vi "Set Properties from Cluster.vi"(8 "error in":errorcluster, 10 "Variant Cluster":variant, 11 "item ref in":T1 format="%.0x") -> (0 "error out":errorcluster, 3 "item ref out":T1 format="%.0x")   [LabVIEW 2020, in "AIM ARINC 664 Scripting.lvlib"]
doc: "Set the parameters cluster into the system definition, separating each element by name in cluster.\n\nBe sure that cluster element names are matching Veristand Property names.\n\nDo not pass clusters of clusters or array of cluster as inputs to this VI. It only works with plain clusters."
uses:
  AIM ARINC 664 Scripting.lvlib
  <vilib>/NI VeriStand/Custom Device API/Custom Device Item Ref.ctl
  <vilib>/NI VeriStand/Custom Device API/Set Item Property (U32).vi
  <vilib>/NI VeriStand/Custom Device API/Set Item Property (U16).vi
  <vilib>/NI VeriStand/Custom Device API/Set Item Property (Double).vi
  <vilib>/NI VeriStand/Custom Device API/Set Item Property (I32).vi
  <vilib>/NI VeriStand/Custom Device API/Set Item Property (String).vi
  <vilib>/NI VeriStand/Custom Device API/Set Item Property (Path).vi
  <vilib>/NI VeriStand/Custom Device API/Set Item Property (Boolean).vi
  <vilib>/NI VeriStand/Custom Device API/Custom Device API.lvlib
  <vilib>/Utility/Data Type/NI_Data Type.lvlib
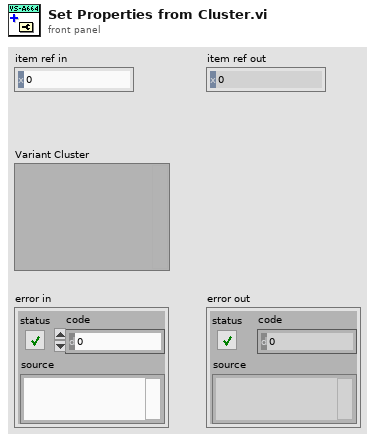
[diagram p1: front panel]
types:
  T1 = typedef "Custom Device API.lvlib/Custom Device Item Ref.ctl" = u64
  T2 = typedef "NI_Data Type.lvlib/Data Type.ctl" = enum8{"Invalid Type", "Void", "I8", "I16", "I32", "I64", "U8", "U16", "U32", "U64", "Single Float", "Double Float", "Extended Float", "Single Complex", "Double Complex", "Extended Complex", "Enum U8", "Enum U16", "Enum U32", "Enum U64", "Single Float With Unit", "Double Float With Unit", "Extended Float With Unit", "Single Complex with Unit", "Double Complex with Unit", "Extended Complex with Unit", "Boolean", "String", "Path", "Picture", "Tag", "Array", "Cluster", "Variant", "LV Variant", "Waveform", "Timestamp", "Digital Waveform", "Digital Data", "ExpressData", "Refnum", "External Data", "VI", "Poly VI", "LabVIEW Class Instance", "Fixed Point", "Set Collection", "Map Collection"}
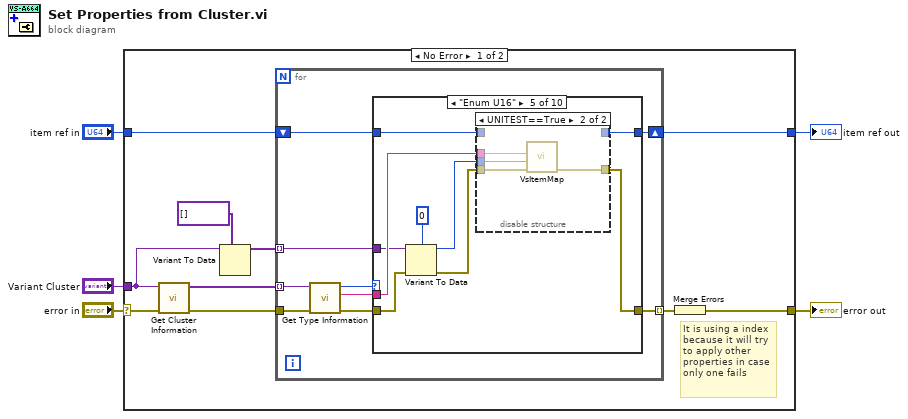
[diagram p0: block diagram]
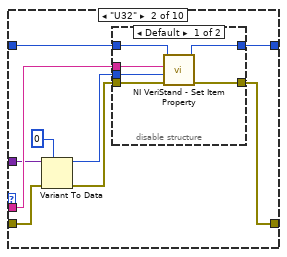
[diagram p3: hidden frame]
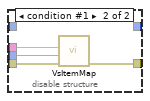
[diagram p4: hidden frame]
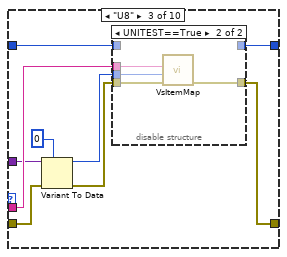
[diagram p5: hidden frame]
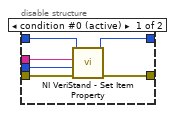
[diagram p6: hidden frame]
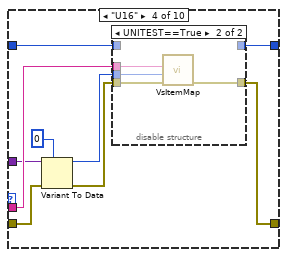
[diagram p7: hidden frame]
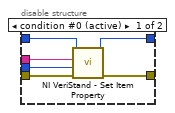
[diagram p8: hidden frame]
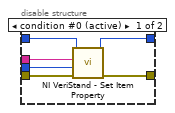
[diagram p9: hidden frame]
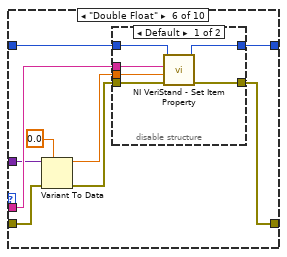
[diagram p10: hidden frame]
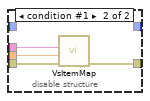
[diagram p11: hidden frame]
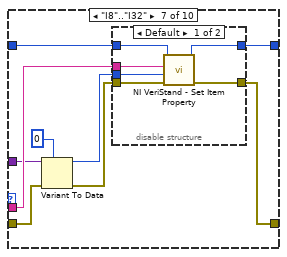
[diagram p12: hidden frame]
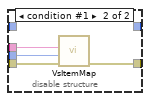
[diagram p13: hidden frame]
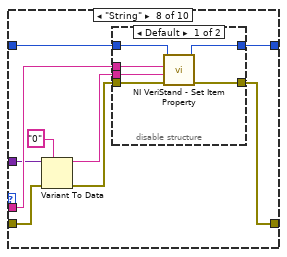
[diagram p14: hidden frame]
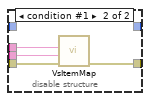
[diagram p15: hidden frame]
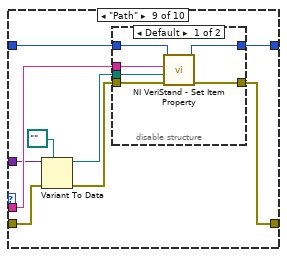
[diagram p16: hidden frame]
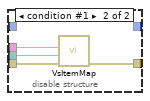
[diagram p17: hidden frame]
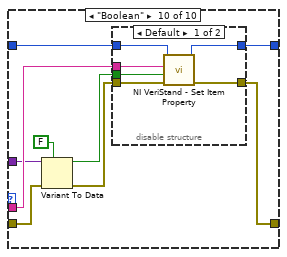
[diagram p18: hidden frame]
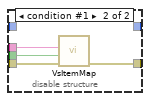
[diagram p19: hidden frame]
diagram:
  n1 = case shown="No Error" "error in" {
    selector: "error in" -> [w6 w190]
    tunnel: "item ref in" -> [w15 w189]
    tunnel: [w13 w189] -> w4
    tunnel: "Variant Cluster" -> [w8 _]
    tunnel: [w7 w190] -> w2
    frame No Error {
      # "It is using a index\nbecause it will try\nto apply other\nproperties in case\nonly one fails"
      n2 = call <vilib>:"Get Cluster Information.vi"("error in (no error)"=w6, "variant"=w8) -> ("error out"=w11:errorcluster, "cluster elements"=w12:variant[])  [unwired: 8 in]
      n3 = Variant To Data(type=variant[] [], Variant=w8) -> (data=w10:variant[])  [unwired: 1 in, 1 out]
      n4 = for {
        tunnel: w12 -> [w24] mode=indexing
        shift-right: [w20] -> w13
        shift-left: w15 -> [w21]
        tunnel: w10 -> [w16] mode=indexing
        tunnel: w11 -> [w23]
        tunnel: [w17] -> w14 mode=indexing
        n5 = call <vilib>:"Get Type Information.vi"("error in (no error)"=w23, "variant"=w24) -> ("error out"=w18:errorcluster, "name"=w22:string, "type"=w19:T2)  [unwired: 5 in, 2 out]
        n6 = case shown="\"Enum U16\"" w19 {
          tunnel: w22 -> [_ w35 w53 w71 w89 w107 w125 w143 w161 w179]
          tunnel: w21 -> [w26 w34 w52 w70 w88 w106 w124 w142 w160 w178]
          tunnel: [w26 w33 w51 w69 w87 w105 w123 w141 w159 w177] -> w20
          tunnel: w18 -> [w25 w28 w46 w64 w83 w100 w118 w136 w154 w173]
          tunnel: [w25 w32 w50 w68 w86 w104 w122 w140 w158 w176] -> w17
          tunnel: w16 -> [_ w31 w49 w67 w85 w103 w121 w139 w157 w175]
          frame "Invalid Type", Default {
          }
          frame "U32" {
            n7 = Variant To Data(error in=w28, type=u32 0, Variant=w31) -> (data=w30:u32, error out=w27:errorcluster)
            n8 = disable-structure shown="Default" {
              disable-tunnel: w35 -> [w41 w44]
              disable-tunnel: w34 -> [w40 _]
              disable-tunnel: [w39 _] -> w33
              disable-tunnel: [w38 w42] -> w32
              disable-tunnel: w30 -> [w37 w43]
              disable-tunnel: w27 -> [w36 w42]
              frame condition #0 (active) {
                n9 = call-poly <vilib>:"NI VeriStand - Set Item Property.vi"("error in (no error)"=w36, "Value"=w37, "Property Name"=w41, "Item Ref in"=w40) -> ("error out"=w38:errorcluster, "Item Ref out"=w39:T1)  [unwired: 5 in, 1 out]
              }
              frame condition #1 {
                n10 = call "VsItemMap.vi"("Variant"=w43, "name"=w44) -> ()  [unwired: 9 in, 1 out]
              }
            }
          }
          frame "U8" {
            n11 = Variant To Data(error in=w46, type=u8 0, Variant=w49) -> (data=w48:u8, error out=w45:errorcluster)
            n12 = disable-structure shown="UNITEST==True" {
              disable-tunnel: w53 -> [w59 w62]
              disable-tunnel: w52 -> [w58 _]
              disable-tunnel: [w57 _] -> w51
              disable-tunnel: [w56 w60] -> w50
              disable-tunnel: w48 -> [w55 w61]
              disable-tunnel: w45 -> [w54 w60]
              frame condition #0 (active) {
                n13 = call-poly <vilib>:"NI VeriStand - Set Item Property.vi"("error in (no error)"=w54, "Value"=w55, "Property Name"=w59, "Item Ref in"=w58) -> ("error out"=w56:errorcluster, "Item Ref out"=w57:T1)  [unwired: 5 in, 1 out]
              }
              frame condition #1 {
                n14 = call "VsItemMap.vi"("Variant"=w61, "name"=w62) -> ()  [unwired: 9 in, 1 out]
              }
            }
          }
          frame "U16" {
            n15 = Variant To Data(error in=w64, type=u16 0, Variant=w67) -> (data=w66:u16, error out=w63:errorcluster)
            n16 = disable-structure shown="UNITEST==True" {
              disable-tunnel: w71 -> [w77 w80]
              disable-tunnel: w70 -> [w76 _]
              disable-tunnel: [w75 _] -> w69
              disable-tunnel: [w74 w78] -> w68
              disable-tunnel: w66 -> [w73 w79]
              disable-tunnel: w63 -> [w72 w78]
              frame condition #0 (active) {
                n17 = call-poly <vilib>:"NI VeriStand - Set Item Property.vi"("error in (no error)"=w72, "Value"=w73, "Property Name"=w77, "Item Ref in"=w76) -> ("error out"=w74:errorcluster, "Item Ref out"=w75:T1)  [unwired: 5 in, 1 out]
              }
              frame condition #1 {
                n18 = call "VsItemMap.vi"("Variant"=w79, "name"=w80) -> ()  [unwired: 9 in, 1 out]
              }
            }
          }
          frame "Enum U16" {
            n19 = Variant To Data(error in=w83, type=u16 0, Variant=w85) -> (data=w84:u16, error out=w82:errorcluster)
            n20 = disable-structure shown="UNITEST==True" {
              disable-tunnel: w89 -> [w95 w98]
              disable-tunnel: w88 -> [w94 _]
              disable-tunnel: [w93 _] -> w87
              disable-tunnel: [w92 w96] -> w86
              disable-tunnel: w84 -> [w91 w97]
              disable-tunnel: w82 -> [w90 w96]
              frame condition #0 (active) {
                n21 = call-poly <vilib>:"NI VeriStand - Set Item Property.vi"("error in (no error)"=w90, "Value"=w91, "Property Name"=w95, "Item Ref in"=w94) -> ("error out"=w92:errorcluster, "Item Ref out"=w93:T1)  [unwired: 5 in, 1 out]
              }
              frame condition #1 {
                n22 = call "VsItemMap.vi"("Variant"=w97, "name"=w98) -> ()  [unwired: 9 in, 1 out]
              }
            }
          }
          frame "Double Float" {
            n23 = Variant To Data(error in=w100, type=0.0, Variant=w103) -> (data=w102:dbl, error out=w99:errorcluster)
            n24 = disable-structure shown="Default" {
              disable-tunnel: w107 -> [w113 w116]
              disable-tunnel: w106 -> [w112 _]
              disable-tunnel: [w111 _] -> w105
              disable-tunnel: [w110 w114] -> w104
              disable-tunnel: w102 -> [w109 w115]
              disable-tunnel: w99 -> [w108 w114]
              frame condition #0 (active) {
                n25 = call-poly <vilib>:"NI VeriStand - Set Item Property.vi"("error in (no error)"=w108, "Value"=w109, "Property Name"=w113, "Item Ref in"=w112) -> ("error out"=w110:errorcluster, "Item Ref out"=w111:T1)  [unwired: 5 in, 1 out]
              }
              frame condition #1 {
                n26 = call "VsItemMap.vi"("Variant"=w115, "name"=w116) -> ()  [unwired: 9 in, 1 out]
              }
            }
          }
          frame "I8".."I32" {
            n27 = Variant To Data(error in=w118, type=0, Variant=w121) -> (data=w120:i32, error out=w117:errorcluster)
            n28 = disable-structure shown="Default" {
              disable-tunnel: w125 -> [w131 w134]
              disable-tunnel: w124 -> [w130 _]
              disable-tunnel: [w129 _] -> w123
              disable-tunnel: [w128 w132] -> w122
              disable-tunnel: w120 -> [w127 w133]
              disable-tunnel: w117 -> [w126 w132]
              frame condition #0 (active) {
                n29 = call-poly <vilib>:"NI VeriStand - Set Item Property.vi"("error in (no error)"=w126, "Value"=w127, "Property Name"=w131, "Item Ref in"=w130) -> ("error out"=w128:errorcluster, "Item Ref out"=w129:T1)  [unwired: 5 in, 1 out]
              }
              frame condition #1 {
                n30 = call "VsItemMap.vi"("Variant"=w133, "name"=w134) -> ()  [unwired: 9 in, 1 out]
              }
            }
          }
          frame "String" {
            n31 = Variant To Data(error in=w136, type="0", Variant=w139) -> (data=w138:string, error out=w135:errorcluster)
            n32 = disable-structure shown="Default" {
              disable-tunnel: w143 -> [w149 w152]
              disable-tunnel: w142 -> [w148 _]
              disable-tunnel: [w147 _] -> w141
              disable-tunnel: [w146 w150] -> w140
              disable-tunnel: w138 -> [w145 w151]
              disable-tunnel: w135 -> [w144 w150]
              frame condition #0 (active) {
                n33 = call-poly <vilib>:"NI VeriStand - Set Item Property.vi"("error in (no error)"=w144, "Value"=w145, "Property Name"=w149, "Item Ref in"=w148) -> ("error out"=w146:errorcluster, "Item Ref out"=w147:T1)  [unwired: 5 in, 1 out]
              }
              frame condition #1 {
                n34 = call "VsItemMap.vi"("Variant"=w151, "name"=w152) -> ()  [unwired: 9 in, 1 out]
              }
            }
          }
          frame "Path" {
            n35 = Variant To Data(error in=w154, type=path "", Variant=w157) -> (data=w156:path, error out=w153:errorcluster)
            n36 = disable-structure shown="Default" {
              disable-tunnel: w161 -> [w167 w170]
              disable-tunnel: w160 -> [w166 _]
              disable-tunnel: [w165 _] -> w159
              disable-tunnel: [w164 w168] -> w158
              disable-tunnel: w156 -> [w163 w169]
              disable-tunnel: w153 -> [w162 w168]
              frame condition #0 (active) {
                n37 = call-poly <vilib>:"NI VeriStand - Set Item Property.vi"("error in (no error)"=w162, "Value"=w163, "Property Name"=w167, "Item Ref in"=w166) -> ("error out"=w164:errorcluster, "Item Ref out"=w165:T1)  [unwired: 5 in, 1 out]
              }
              frame condition #1 {
                n38 = call "VsItemMap.vi"("Variant"=w169, "name"=w170) -> ()  [unwired: 9 in, 1 out]
              }
            }
          }
          frame "Boolean" {
            n39 = Variant To Data(error in=w173, type=FALSE, Variant=w175) -> (data=w174:bool, error out=w172:errorcluster)
            n40 = disable-structure shown="Default" {
              disable-tunnel: w179 -> [w185 w188]
              disable-tunnel: w178 -> [w184 _]
              disable-tunnel: [w183 _] -> w177
              disable-tunnel: [w182 w186] -> w176
              disable-tunnel: w174 -> [w181 w187]
              disable-tunnel: w172 -> [w180 w186]
              frame condition #0 (active) {
                n41 = call-poly <vilib>:"NI VeriStand - Set Item Property.vi"("error in (no error)"=w180, "Value"=w181, "Property Name"=w185, "Item Ref in"=w184) -> ("error out"=w182:errorcluster, "Item Ref out"=w183:T1)  [unwired: 5 in, 1 out]
              }
              frame condition #1 {
                n42 = call "VsItemMap.vi"("Variant"=w187, "name"=w188) -> ()  [unwired: 9 in, 1 out]
              }
            }
          }
        }
      }
      n43 = Merge Errors(w14) -> (w7:errorcluster)
    }
    frame Error {
      # "Propagate the \"error in\" properly"
    }
  }
  "error out" <- w2
  "item ref out" <- w4
